vi "UDSOpenSession.vi"(8 "error in (no error)":errorcluster, 11 "UDS Session Parameters":T6 {"Receive ID" format="%x"; "Transmit ID" format="%x"}) -> (0 "error out":errorcluster, 3 "UDS Session Out":T1={"Diag CAN Handle"=0, "Transport Protocol"=enum."ISO TP - Normal Mode", "Receive Address Extension"=0, "Transmit Address Extension"=0, "Receive CAN Id"=0, "Transmit CAN Id"=0, "Log Frames ?"=FALSE, "My TP Address"=0, "Other TP Address"=0, "T1"=0, "T2"=0, "T3"=0, "T4"=0, "Tx SN"=0, "Block Size"=0, "Rx SN"=0, "VW TP Initialized?"=FALSE, "Tx block no"=0, "baud rate"=0, "Interface"="", "Channel Diag CAN Handle"=0, "UDP Connection ID"=refnum, "TCP Connection ID"=refnum, "Target IP Addr"=0, "Source Address"=0, "Target Address"=0, "Send Header NACK?"=FALSE, "DLL Handle"=0, "NAD"=0, "Time Stamp read first"=0.0, "Time Stamp read last"=0.0, "Time Stamp write first"=0.0, "Time Stamp write last"=0.0, "Time Stamp write"=0.0, "Time Stamp read"=0.0, " I/O Mode"=0, "FD Baudrate"=1000000, "TX_DL"=8, "RX_DL"=8, "DoIP Protocol Version"=1, " Selected I/O Mode"=0, "TesterPresent Counter"=0, "TesterPresent Limit"=0, "TesterPresent Tick[ms]"=10, "TesterPresent RequireResponse?"=FALSE, "TesterPresent Stored Ref?"=FALSE, "TesterPresent Message"=[], "TesterPresent Task Handle"=0, "TesterPresent Semaphore"=refnum, "Response Plausibility Check"=1, "Default Version?"=TRUE, "Diagostic Globals"={"Timeout FC (Bs)"=250, "Timeout CF (Cr)"=250, "Timeout Diag Command"=1000, "Receive Block Size (BS)"=232, "Wait Time CF (STmin)"=232, "Max Waits (N_WFTmax)"=232, "Waits to Send (N_WAIT)"=232, "Time between Waits (TW)"=232, "Fill CAN Frames?"=FALSE, "Fill Byte"=0, "Invalid Response as Error?"=FALSE, "Max RspPending Count"=5, "VWTP Command Timeout"=50, "Transport Protocol"=enum."ISO TP - Normal Mode", "Diag CAN Handle"=0, "DLL Handle"=0, "Timeout RspPending"=1000}, "Session-based Properties?"=FALSE, "NI-XNET IP Stack Reference"=0, "NI-XNET IP Stack TCP Reference"=-1, "NI-XNET IP Stack UDP Reference"=-1, "NI-XNET IP Stack Local Interface"="", "Functional CAN Id"=0, "Diag CAN Queue"=refnum, "Frame Fillling Mode"=0, "DoIP Acknowledge Mode"=0, "Message Buffer"=[]} {"Diagostic Globals"."Fill Byte" format="%x"; "TesterPresent Message" format="%.0x"; "Selected I/O Mode" items=["CAN", "CAN FD", "CAN FD+BRS", "ECU Determined"]; "DoIP Protocol Version" items=["2010"=1, "2012"=2]; "RX_DL" items=["8"=8, "12"=12, "16"=16, "20"=20, "24"=24, "32"=32, "48"=48, "64"=64]; "TX_DL" items=["8"=8, "12"=12, "16"=16, "20"=20, "24"=24, "32"=32, "48"=48, "64"=64]; "I/O Mode" items=["CAN", "CAN FD", "CAN FD+BRS", "Not yet determined"]})   [LabVIEW 2021, in "Lunar UDS CAN.lvlib"]
uses:
  Lunar UDS CAN.lvlib
  Controls/UDSSessionParameters.ctl
  <vilib>/Automotive Diagnostic Command Set/Diagnostic Transport.llb/Diag Reference.ctl
  <vilib>/Automotive Diagnostic Command Set/Diagnostic Transport.llb/Transport Protocol Selector.ctl
  <vilib>/Automotive Diagnostic Command Set/Diagnostic Transport.llb/DoIP Protocol Version.ctl
  <vilib>/Automotive Diagnostic Command Set/Diagnostic Transport.llb/Diag Globals.ctl
  <vilib>/Automotive Diagnostic Command Set/Diagnostic Transport.llb/Property ID.ctl
  <vilib>/addons/Automotive Diagnostic Command Set/NI_Automotive Diagnostic Command Set.lvlib
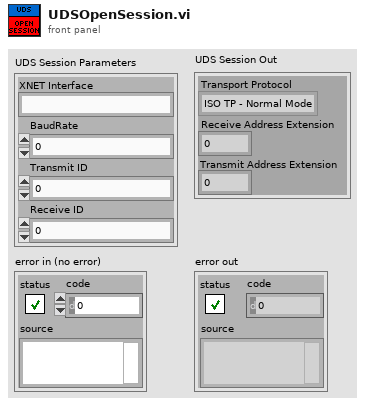
[diagram p1: front panel]
types:
  T1 = typedef "NI_Automotive Diagnostic Command Set.lvlib/Diag Reference.ctl" = cluster{"Diag CAN Handle":u32, "Transport Protocol":T2, "Receive Address Extension":u8, "Transmit Address Extension":u8, "Receive CAN Id":u32, "Transmit CAN Id":u32, "Log Frames ?":bool, "My TP Address":u8, "Other TP Address":u8, "T1":u16, "T2":u16, "T3":u16, "T4":u16, "Tx SN":u8, "Block Size":u8, "Rx SN":u8, "VW TP Initialized?":bool, "Tx block no":u8, "baud rate":u64, "Interface":string, "Channel Diag CAN Handle":u32, "UDP Connection ID":refnum<k16>, "TCP Connection ID":refnum<k5>, "Target IP Addr":u32, "Source Address":u16, "Target Address":u16, "Send Header NACK?":bool, "DLL Handle":u32, "NAD":u8, "Time Stamp read first":dbl, "Time Stamp read last":dbl, "Time Stamp write first":dbl, "Time Stamp write last":dbl, "Time Stamp write":dbl, "Time Stamp read":dbl, " I/O Mode":u32, "FD Baudrate":u64, "TX_DL":u16, "RX_DL":u16, "DoIP Protocol Version":T3, " Selected I/O Mode":u32, "TesterPresent Counter":u32, "TesterPresent Limit":u32, "TesterPresent Tick[ms]":i32, "TesterPresent RequireResponse?":bool, "TesterPresent Stored Ref?":bool, "TesterPresent Message":u8[], "TesterPresent Task Handle":i32, "TesterPresent Semaphore":T4, "Response Plausibility Check":u32, "Default Version?":bool, "Diagostic Globals":T5, "Session-based Properties?":bool, "NI-XNET IP Stack Reference":i64, "NI-XNET IP Stack TCP Reference":i64, "NI-XNET IP Stack UDP Reference":i64, "NI-XNET IP Stack Local Interface":string, "Functional CAN Id":u32, "Diag CAN Queue":refnum<queue>, "Frame Fillling Mode":u32, "DoIP Acknowledge Mode":u32, "Message Buffer":u8[]}
  T2 = typedef "NI_Automotive Diagnostic Command Set.lvlib/Transport Protocol Selector.ctl" = enum16{"ISO TP - Normal Mode", "ISO TP - Mixed Mode", "VW TP 2.0", "Diagnostics on IP", "ISO TP LIN"}
  T3 = typedef "NI_Automotive Diagnostic Command Set.lvlib/DoIP Protocol Version.ctl" = u8
  T4 = typedef "Semaphore RefNum" = refnum<k1>
  T5 = typedef "NI_Automotive Diagnostic Command Set.lvlib/Diag Globals.ctl" = cluster{"Timeout FC (Bs)":u32, "Timeout CF (Cr)":u32, "Timeout Diag Command":u32, "Receive Block Size (BS)":u8, "Wait Time CF (STmin)":u8, "Max Waits (N_WFTmax)":u8, "Waits to Send (N_WAIT)":i32, "Time between Waits (TW)":u32, "Fill CAN Frames?":bool, "Fill Byte":u32, "Invalid Response as Error?":bool, "Max RspPending Count":u32, "VWTP Command Timeout":u32, "Transport Protocol":T2, "Diag CAN Handle":u32, "DLL Handle":u32, "Timeout RspPending":u32}
  T6 = typedef "Lunar UDS CAN.lvlib/UDSSessionParameters.ctl" = cluster{"XNET Interface":string, "BaudRate":u64, "Transmit ID":i32, "Receive ID":i32}
  T7 = typedef "NI_Automotive Diagnostic Command Set.lvlib/Property ID.ctl" = enum16{"Timeout Diag Command", "Timeout FC (Bs)", "Timeout CF (Cr)", "Receive Block Size (BS)", "Wait Time CF (STmin)", "Max Wait Frames (N_WFTmax)", "Wait Frames to Send (N_WAIT)", "Time between Waits (T_W)", "Fill CAN Frames", "Fill Byte", "Invalid Response as Error", "Max RspPending Count", "VWTP Command Timeout", "STmin", "P2min", "Termination", "Timeout RspPending", "LIN Sleep", "Actual CAN IO Mode", "Response Plausibility Check", "Session-based Properties", "DoIP Acknowledge Mode"}
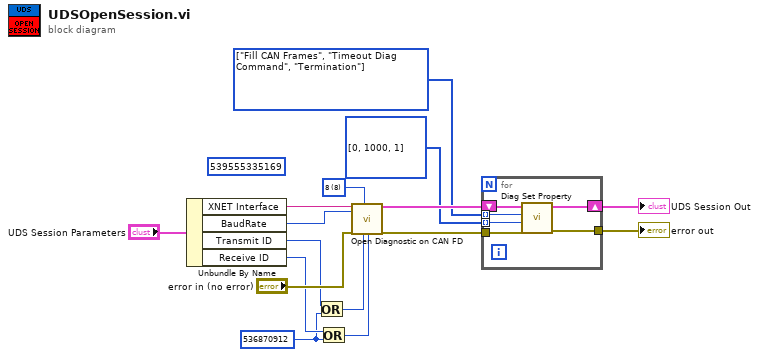
[diagram p0: block diagram]
diagram:
  (unwired) u64 539555335169 ("Baud Rate")
  w2 = T7[] [enum."Fill CAN Frames", enum."Timeout Diag Command", enum."Termination"] items=["Timeout Diag Command", "Timeout FC (Bs)", "Timeout CF (Cr)", "Receive Block Size (BS)", "Wait Time CF (STmin)", "Max Wait Frames (N_WFTmax)", "Wait Frames to Send (N_WAIT)", "Time between Waits (T_W)", "Fill CAN Frames", "Fill Byte", "Invalid Response as Error", "Max RspPending Count", "VWTP Command Timeout", "STmin", "P2min", "Termination", "Timeout RspPending", "LIN Sleep", "Actual CAN IO Mode", "Response Plausibility Check", "Session-based Properties", "DoIP Acknowledge Mode"]
  w8 = u16 8 items=["8"=8, "12"=12, "16"=16, "20"=20, "24"=24, "32"=32, "48"=48, "64"=64] ("Max DLC")
  w11 = 536870912
  n1 = Unbundle By Name("UDS Session Parameters") -> ("XNET Interface"=w14:string, "BaudRate"=w1:u64, "Transmit ID"=w13:i32, "Receive ID"=w12:i32)
  n2 = Or(x=w13, y=w11) -> (x .or. y?=w10:i32)
  n3 = Or(x=w12, y=w11) -> (x .or. y?=w9:i32)
  n4 = call <vilib>:"Open Diagnostic on CAN FD.vi"("CAN Interface"=w14, "Baud Rate"=w1, "error in (no error)"="error in (no error)", "Max DLC"=w8, "Transmit ID"=w10, "Receive ID"=w9) -> ("diag ref out"=w4:T1, "error out"=w7:errorcluster)  [unwired: 12 in]
  n5 = for {
    tunnel: w7 -> [w22]
    tunnel: [w21] -> w6
    shift-right: [w20] -> w5
    shift-left: w4 -> [w19]
    tunnel: i32[] [0, 1000, 1] -> [w18] mode=indexing
    tunnel: w2 -> [w17] mode=indexing
    n6 = call <vilib>:"Diag Set Property.vi"("error in (no error)"=w22, "property value"=w18, "property ID"=w17, "diag ref in"=w19) -> ("error out"=w21:errorcluster, "diag ref out"=w20:T1)  [unwired: 6 in]
  }
  "error out" <- w6
  "UDS Session Out" <- w5
